vi "POV Protection.vi"(1 "Array":i16[](array[numeric])) -> (0 "s? t:f":i32)   [LabVIEW 2018]
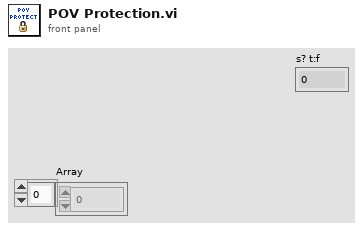
[diagram p1: front panel]
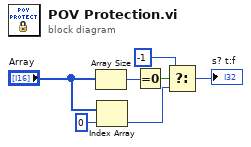
[diagram p0: block diagram]
diagram:
  n1 = Array Size(array="Array") -> (size(s)=w7:i32)
  n2 = Index Array(array="Array", index=0) -> (element=w2:i16)
  n3 = Equal To 0?(x=w7) -> (x = 0?=w6:bool)
  n4 = Select(t=-1, s=w6, f=w2) -> (s? t:f=→"s? t:f":i32)
